vi "Main.vi"(10 "Monedas Subpanel":refnum<vi>, 11 "Module Admin":refnum<class "Delacor_lib_QMH_Module Admin.lvclass">) -> ()   [LabVIEW 2020, in "Monedas.lvlib"]
doc: "This template is based off of the Queued Message Handler design pattern and the Queued Message Handler project template that ships with LabVIEW.\n\nThe main difference is that the queue is private to this module and communication between modules is performed via Broadcast and Request events.\n\nRequest events are wrapped in public API methods and are handled in the Event Handling Loop (EHL) of this VI. Any module can register for Broadcast events sent by this module. The EHL generates messages based on user interface actions.\n\nThe Message Handling Loop (MHL) processes messages generated by the EHL, or by other messages. The messages are string values, so new messages can be added easily to the Message Cases case structure in the MHL. Each message cluster can also provide an optional value for Message Data, which is a variant that can be converted to whatever message-specific data is required.\n_____\nBased on Delacor QMH Project Template 5.0.0.82."
uses:
  Monedas.lvlib
  <vilib>/Delacor/Delacor QMH/Libraries/Module Admin_class/Delacor_lib_QMH_Module Admin.lvclass
  Module Data--cluster.ctl
  Stop Argument--cluster.ctl
  <vilib>/Delacor/Delacor QMH/Libraries/Message Queue_class/Delacor_lib_QMH_Message Queue.lvclass/Delacor_lib_QMH_Message Queue.ctl
  <vilib>/Delacor/Delacor QMH/Libraries/Module Admin_class/Delacor_lib_QMH_Module Admin.lvclass/Delacor_lib_QMH_Module Admin.ctl
  Coin pressed Argument--cluster.ctl
  Set coin values Argument--cluster.ctl
  Reset credit to 0 Argument--cluster.ctl
  Ask if credit Argument--cluster.ctl
  Ask if credit (Reply Payload)--cluster.ctl
  <vilib>/Utility/miscctls.llb/LVPointTypeDef.ctl
  <vilib>/Delacor/Delacor QMH/Libraries/Message Queue_class/Delacor_lib_QMH_Enqueue Message (Single).vi
  <vilib>/Delacor/Delacor QMH/Libraries/Module Admin_class/Delacor_lib_QMH_Get External Launch.vi
  <vilib>/Utility/error.llb/Error Cluster From Error Code.vi
  <vilib>/ErrorRing/Error Ring.xnode
  <vilib>/Delacor/Delacor QMH/Libraries/Message Queue_class/Delacor_lib_QMH_Message Queue.lvclass
  Mensajes/Mensajes.lvlib
panel:
  out "Status":string
  in  "Monedas":cluster{"1":bool, "2":bool, "3":bool, "4":bool}
  out "error out":errorcluster
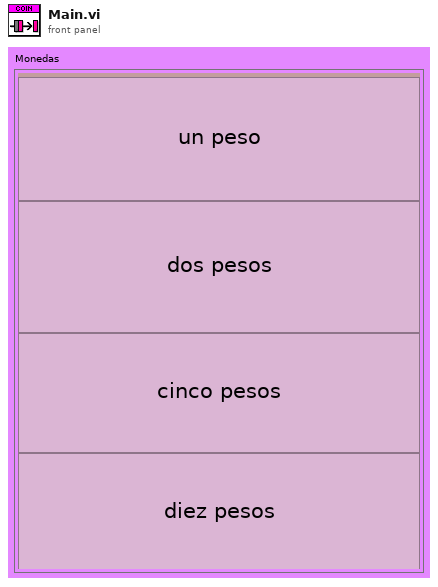
[diagram p1: front panel]
types:
  T1 = typedef "Monedas.lvlib/Request Events--cluster.ctl" = cluster{"Stop Module":refnum<user-event>, "Show Panel":refnum<user-event>, "Hide Panel":refnum<user-event>, "Get Module Execution Status":refnum<user-event>, "Show Diagram":refnum<user-event>, "Coin pressed":refnum<user-event>, "Set coin values":refnum<user-event>, "Request credit":refnum<user-event>, "Reset credit to 0":refnum<user-event>, "Ask if credit":refnum<user-event>}
  T2 = typedef "Monedas.lvlib/Module Data--cluster.ctl" = cluster{"Status":string, "Credit":dbl, "Refs":cluster{"Ref 1":refnum<vi>, "Ref 2":refnum<vi>, "Ref 3":refnum<vi>, "Ref 4":refnum<vi>}, "Coins":cluster{"Boolean Text":string, "Value":i32}[]}
  T3 = enum32{"invalid lock state", "Not Locked", "Locked (No Password)", "Password-protected"}
  T4 = typedef "Monedas.lvlib/Stop Argument--cluster.ctl" = cluster{"Origin":string, "Exit via Stop Module Req?":bool, "Wait for Module to stop?":bool}
  T5 = typedef "Monedas.lvlib/Coin pressed Argument--cluster.ctl" = cluster{"Coin Number":i32}
  T6 = typedef "Monedas.lvlib/Set coin values Argument--cluster.ctl" = cluster{"Coins":cluster{"Boolean Text":string, "Value":i32}[]}
  T7 = typedef "Monedas.lvlib/Reset credit to 0 Argument--cluster.ctl" = cluster{"Boolean":bool}
  T8 = typedef "Monedas.lvlib/Ask if credit Argument--cluster.ctl" = cluster{"Wait Notifier":refnum<notifier>, "wait for reply":bool}
  T9 = typedef "LVPointTypeDef.ctl" = cluster{"Horizontal":i16, "Vertical":i16}
  T10 = enum32{"Invalid", "Standard", "Closed", "Hidden", "Minimized", "Maximized"}
  T11 = typedef "Monedas.lvlib/Ask if credit (Reply Payload)--cluster.ctl" = cluster{"Credit":dbl, "Ask if credit_error":errorcluster}
  T12 = cluster{"Ref 1":refnum<vi>, "Ref 2":refnum<vi>, "Ref 3":refnum<vi>, "Ref 4":refnum<vi>}
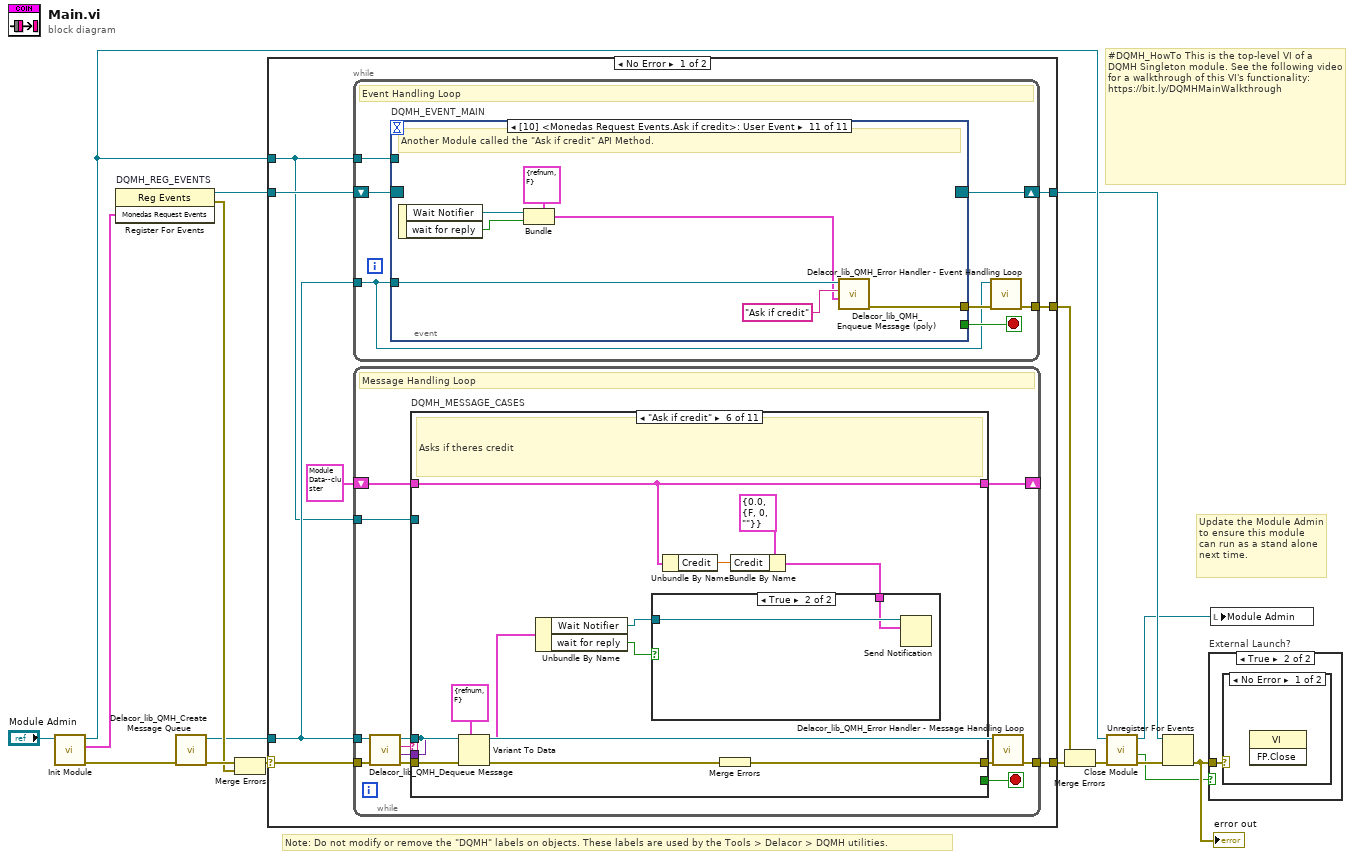
[diagram p0: block diagram]
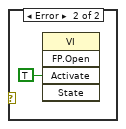
[diagram p3: hidden frame]
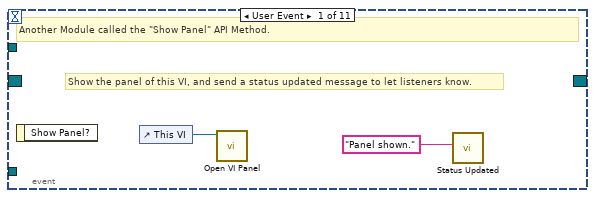
[diagram p4: hidden frame]
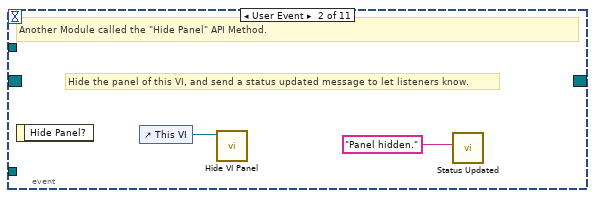
[diagram p5: hidden frame]
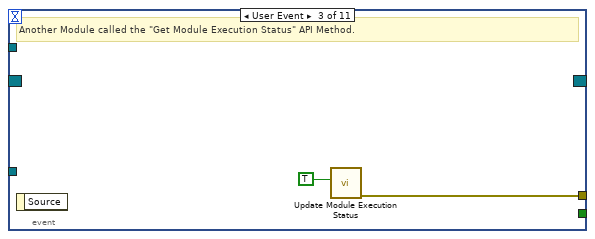
[diagram p6: hidden frame]
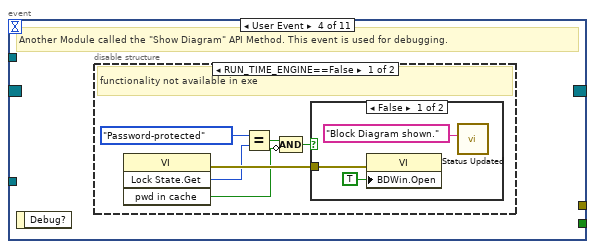
[diagram p7: hidden frame]
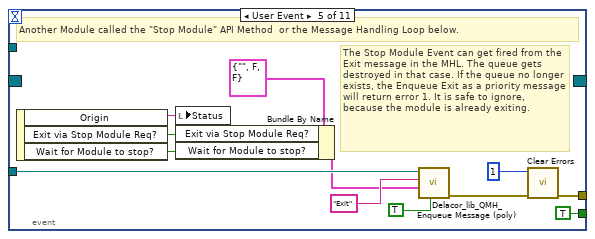
[diagram p10: hidden frame]
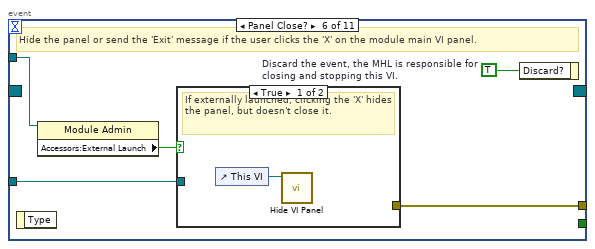
[diagram p11: hidden frame]
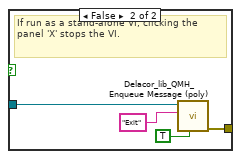
[diagram p12: hidden frame]
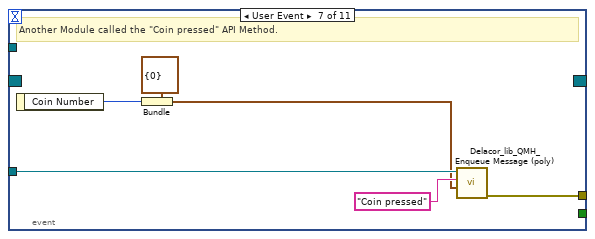
[diagram p13: hidden frame]
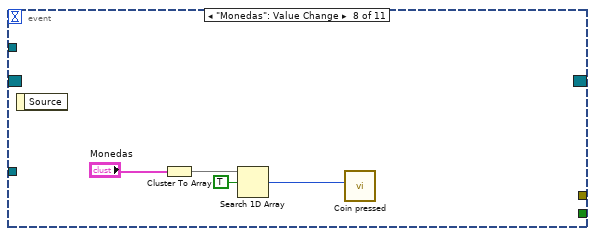
[diagram p14: hidden frame]
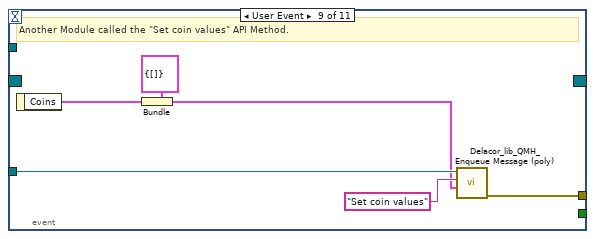
[diagram p15: hidden frame]
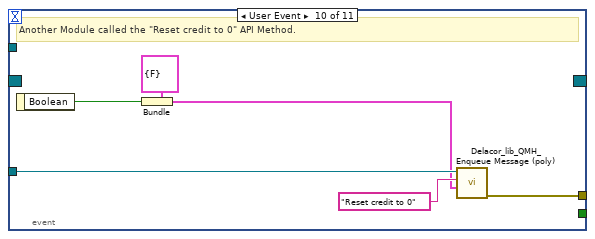
[diagram p16: hidden frame]
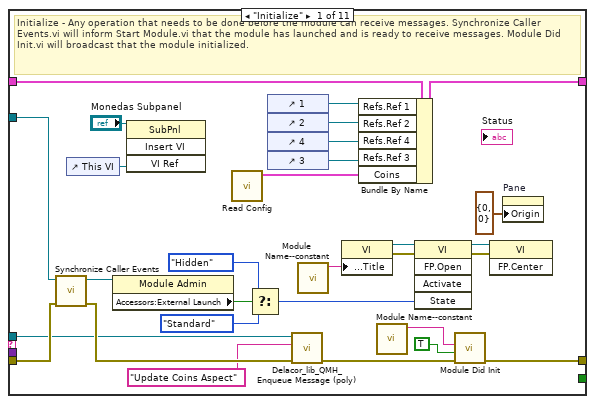
[diagram p17: hidden frame]
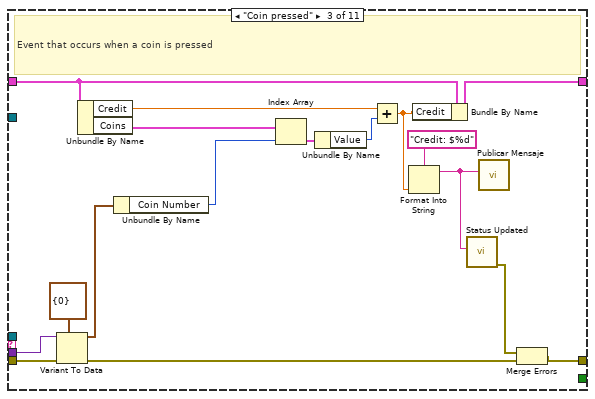
[diagram p19: hidden frame]
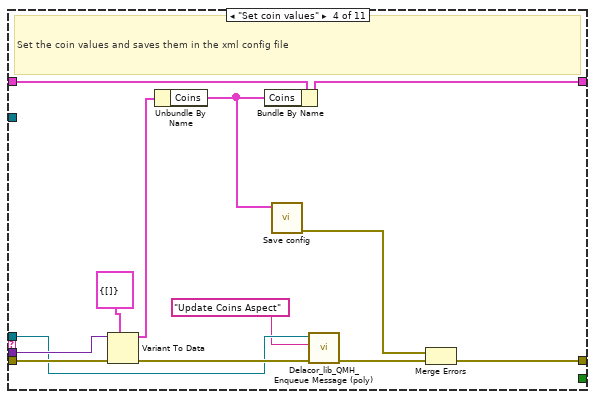
[diagram p20: hidden frame]
diagram:
  # "#DQMH_HowTo This is the top-level VI of a DQMH Singleton module. See the following video for a walkthrough of this VI's functionality: https://bit.ly/DQMHMainWalkthrough"
  # "Note: Do not modify or remove the \"DQMH\" labels on objects. These labels are used by the Tools > Delacor > DQMH utilities."
  # "Update the Module Admin to ensure this module can run as a stand alone next time."
  n1 = call "Init Module.vi"("Singleton Module Admin in"="Module Admin") -> ("error out"=w16:errorcluster, "Monedas Request Events"=w5:T1, "Singleton Module Admin out"=w8:refnum<class "Delacor_lib_QMH_Module Admin.lvclass">)  [unwired: 8 in]
  n2 = register-events "DQMH_REG_EVENTS"(w5) -> (reference out=w6:refnum<event-registration>, error out=w9:errorcluster)  [unwired: 2 in]
  n3 = call <vilib>:"Delacor_lib_QMH_Create Message Queue.vi"("error in (no error)"=w16) -> ("error out"=w11:errorcluster, "Message Queue"=w4:refnum<class "Delacor_lib_QMH_Message Queue.lvclass">)  [unwired: 9 in]
  n4 = Merge Errors(w11, w9) -> (w10:errorcluster)
  n5 = case shown="No Error" w10 {
    selector: w10 -> [w23 w251]
    tunnel: [w25 w250] -> w17
    tunnel: [w22 w256] -> w7
    tunnel: w6 -> [w20 w256]
    tunnel: w4 -> [w19 w249]
    tunnel: [w24 _] -> w14
    tunnel: w8 -> [w18 w252]
    frame No Error {
      n6 = while {
        tunnel: w19 -> [w26]
        shift-right: [w29] -> w22
        shift-left: w20 -> [w30]
        tunnel: [w31] -> w24
        tunnel: w18 -> [w27]
        stop <- w28 stop-if-true
        # "Event Handling Loop"
        n7 = event "DQMH_EVENT_MAIN" shown="[10] <Monedas Request Events.Ask if credit>: User Event" {
          selector: w30 -> [_ _ _ _ _ _ _ _ _ _ _]
          dyn-events: [_ _ _ _ _ _ _ _ _ _ _] -> w29
          timeout: _ -> [_ _ _ _ _ _ _ _ _ _ _]
          tunnel: [_ _ _ _ TRUE ("Discard?") _ _ _ _ _ _] -> w28
          tunnel: w26 -> [_ _ _ _ w55 w62 w75 _ w85 w91 w98]
          tunnel: [_ _ w38 _ w58 w64 w71 _ w80 w86 w92] -> w32
          tunnel: w27 -> [_ _ _ _ _ w61 _ _ _ _ _]
          event User Event {
            # "Show the panel of this VI, and send a status updated message to let listeners know."
            # "Another Module called the \"Show Panel\" API Method."
            n8 = event-data() -> ()  [unwired: 1 in, 1 out]
            n9 = control-ref of="This VI"() -> (w34:refnum<vi>)
            n10 = call "Open VI Panel.vi"("VI"=w34) -> ()  [unwired: 10 in, 1 out]
            n11 = call "Status Updated.vi"("Status"="Panel shown." ("format string")) -> ()  [unwired: 10 in, 1 out]
          }
          event User Event {
            # "Hide the panel of this VI, and send a status updated message to let listeners know."
            # "Another Module called the \"Hide Panel\" API Method."
            n12 = event-data() -> ()  [unwired: 1 in, 1 out]
            n13 = control-ref of="This VI"() -> (w36:refnum<vi>)
            n14 = call "Hide VI Panel.vi"("VI"=w36) -> ()  [unwired: 10 in, 1 out]
            n15 = call "Status Updated.vi"("Status"="Panel hidden." ("format string")) -> ()  [unwired: 10 in, 1 out]
          }
          event User Event {
            # "Another Module called the \"Get Module Execution Status\" API Method."
            n16 = event-data() -> ()  [unwired: 1 in, 1 out]
            n17 = call "Update Module Execution Status.vi"("Running?"=TRUE) -> ("error out"=w38:errorcluster)  [unwired: 10 in]
          }
          event User Event {
            # "Another Module called the \"Show Diagram\" API Method. This event is used for debugging."
            n18 = event-data() -> ()  [unwired: 1 in, 1 out]
            n19 = disable-structure shown="RUN_TIME_ENGINE==False" {
              frame condition #0 (active) {
                # "functionality not available in exe"
                n20 = invoke class="VI" method="Lock State.Get"() -> (error out=w44:errorcluster, "Get Lock State"=w43:T3, "pwd in cache"=w40:bool)  [unwired: 4 in, 1 out]
                n21 = Equal?(x=T3."Password-protected", y=w43) -> (x = y?=w41:bool)
                n22 = Compound Arithmetic op=AND(w41, invert w40) -> (w39:bool)
                n23 = case shown="False" w39 {
                  tunnel: w44 -> [w47 _]
                  frame False {
                    n24 = property class="VI"(error in=w47, "BDWin.Open"=TRUE ("Block Diagram Window:Open")) -> ()  [unwired: 1 in, 2 out]
                    n25 = call "Status Updated.vi"("Status"="Block Diagram shown." ("format string")) -> ()  [unwired: 10 in, 1 out]
                  }
                  frame True {
                    # "Password-protected VI, and the password is not in the cache. Do not show the diagram."
                  }
                }
              }
              frame condition #1 {
              }
            }
          }
          event User Event {
            # "The Stop Module Event can get fired from the Exit message in the MHL. The queue gets destroyed in that case. If the queue no longer exists, the Enqueue Exit as a priority message will return error 1. It is safe to ignore, because the module is already exiting."
            # "Another Module called the \"Stop Module\" API Method  or the Message Handling Loop below."
            n26 = event-data() -> ("Origin"=w54:string, "Exit via Stop Module Req?"=w50:bool, "Wait for Module to stop?"=w49:bool)  [unwired: 1 in]
            n27 = local write "Status"(w54) -> ()
            n28 = Bundle By Name(cluster=T4 {"Origin"="", "Exit via Stop Module Req?"=FALSE, "Wait for Module to stop?"=FALSE} ("Stop Argument"), "Exit via Stop Module Req?"=w50, "Wait for Module to stop?"=w49) -> (w48:T4)
            n29 = call-poly <vilib>:"Delacor_lib_QMH_Enqueue Message (poly).vi"("Priority Message? (F)"=TRUE, "Message Data"=w48, "Message"="Exit", "Message Queue in"=w55) -> ("error out"=w59:errorcluster)  [unwired: 6 in, 1 out]
            n30 = call <vilib>:"Clear Errors.vi"("error in (no error)"=w59, "specific error code to clear (0: all)"=1) -> ("error out"=w58:errorcluster)  [unwired: 4 in, 1 out]
          }
          event Panel Close? {
            w63 = TRUE  # Discard the event, the MHL is responsible for closing and stopping this VI.
            # "Hide the panel or send the 'Exit' message if the user clicks the 'X' on the module main VI panel."
            n31 = event-data() -> ()  [unwired: 1 in, 1 out]
            n32 = property class="Module Admin"(reference=w61) -> ("Accessors:External Launch"=w60:bool)  [unwired: 1 in, 2 out]
            n33 = case shown="True" w60 {
              tunnel: w62 -> [_ w68]
              tunnel: [_ w69] -> w64
              frame True {
                # "If externally launched, clicking the 'X' hides the panel, but doesn't close it."
                n34 = control-ref of="This VI"() -> (w65:refnum<vi>)
                n35 = call "Hide VI Panel.vi"("VI"=w65) -> ()  [unwired: 10 in, 1 out]
              }
              frame False {
                # "If run as a stand-alone VI, clicking the panel 'X' stops the VI."
                n36 = call-poly <vilib>:"Delacor_lib_QMH_Enqueue Message (poly).vi"("Priority Message? (F)"=TRUE, "Message"="Exit", "Message Queue in"=w68) -> ("error out"=w69:errorcluster)  [unwired: 7 in, 1 out]
              }
            }
            n37 = event-data("Discard?"=w63) -> ()  [unwired: 1 in, 1 out]
          }
          event User Event {
            # "Another Module called the \"Coin pressed\" API Method."
            n38 = event-data() -> ("Coin Number"=w70:i32)  [unwired: 1 in]
            n39 = Bundle(cluster=T5 {"Coin Number"=0} ("Coin pressed Argument"), "Coin Number"=w70) -> (w72:T5)
            n40 = call-poly <vilib>:"Delacor_lib_QMH_Enqueue Message (poly).vi"("Message Data"=w72, "Message"="Coin pressed", "Message Queue in"=w75) -> ("error out"=w71:errorcluster)  [unwired: 7 in, 1 out]
          }
          event "Monedas": Value Change {
            n41 = event-data() -> ()  [unwired: 1 in, 1 out]
            n42 = Cluster To Array(cluster="Monedas") -> (array=w78:bool[])
            n43 = Search 1D Array(1D array=w78, element=TRUE) -> (index of element=w77:i32)  [unwired: 1 in]
            n44 = call "Coin pressed.vi"("Coin Number"=w77) -> ()  [unwired: 10 in, 1 out]
          }
          event User Event {
            # "Another Module called the \"Set coin values\" API Method."
            n45 = event-data() -> ("Coins"=w81:cluster{"Boolean Text":string, "Value":i32}[])  [unwired: 1 in]
            n46 = Bundle(cluster=T6 {"Coins"=[]} ("Set coin values Argument"), "Coins"=w81) -> (w82:T6)
            n47 = call-poly <vilib>:"Delacor_lib_QMH_Enqueue Message (poly).vi"("Message Data"=w82, "Message"="Set coin values", "Message Queue in"=w85) -> ("error out"=w80:errorcluster)  [unwired: 7 in, 1 out]
          }
          event User Event {
            # "Another Module called the \"Reset credit to 0\" API Method."
            n48 = event-data() -> ("Boolean"=w87:bool)  [unwired: 1 in]
            n49 = Bundle(cluster=T7 {"Boolean"=FALSE} ("Reset credit to 0 Argument"), "Boolean"=w87) -> (w88:T7)
            n50 = call-poly <vilib>:"Delacor_lib_QMH_Enqueue Message (poly).vi"("Message Data"=w88, "Message"="Reset credit to 0", "Message Queue in"=w91) -> ("error out"=w86:errorcluster)  [unwired: 7 in, 1 out]
          }
          event User Event {
            # "Another Module called the \"Ask if credit\" API Method."
            n51 = event-data() -> ("Wait Notifier"=w94:refnum<notifier>, "wait for reply"=w93:bool)  [unwired: 1 in]
            n52 = Bundle(cluster=T8 {"Wait Notifier"=refnum, "wait for reply"=FALSE} ("Ask if credit Argument"), "Wait Notifier"=w94, "wait for reply"=w93) -> (w95:T8)
            n53 = call-poly <vilib>:"Delacor_lib_QMH_Enqueue Message (poly).vi"("Message Data"=w95, "Message"="Ask if credit", "Message Queue in"=w98) -> ("error out"=w92:errorcluster)  [unwired: 7 in, 1 out]
          }
        }
        n54 = call-dynamic "Delacor_lib_QMH_Error Handler - Event Handling Loop.vi"("error in (no error)"=w32, "Message Queue in"=w26) -> ("dup error in"=w31:errorcluster)  [unwired: 8 in, 1 out]
      }
      n55 = while {
        tunnel: w19 -> [w101]
        shift-right: [w105] -> _
        shift-left: T2 {"Status"="", "Credit"=0.0, "Refs"={"Ref 1"=refnum, "Ref 2"=refnum, "Ref 3"=refnum, "Ref 4"=refnum}, "Coins"=[]} ("Data Cluster") -> [w106]
        tunnel: w23 -> [w109]
        tunnel: [w107] -> w25
        tunnel: w18 -> [w99]
        stop <- w104 stop-if-true
        # "Message Handling Loop"
        n56 = call-dynamic "Delacor_lib_QMH_Dequeue Message.vi"("error in (no error)"=w109, "Message Queue in"=w101) -> ("error out"=w108:errorcluster, "Message Data"=w102:variant, "Message"=w103:string, "Message Queue out"=w100:refnum<class "Delacor_lib_QMH_Message Queue.lvclass">)  [unwired: 6 in]
        n57 = case "DQMH_MESSAGE_CASES" shown="\"Ask if credit\"" w103 {
          selector: w103 -> [_ _ _ _ _ _ _ _ _ _ w236]
          tunnel: w100 -> [w111 _ _ w163 _ _ _ _ w206 w228 _]
          tunnel: w108 -> [w137 w141 w158 w171 w178 w190 w194 w199 w213 w234 w238]
          tunnel: [w135 w141 w144 w160 w176 w181 w194 w199 w209 w231 w239] -> w110
          tunnel: w106 -> [w126 w140 w153 w166 w177 w180 w193 w198 w208 w227 w237]
          tunnel: [w125 w140 w152 w165 w173 w180 w193 w198 w208 w227 w237] -> w105
          tunnel: [_ _ _ _ _ _ _ _ _ w226 _] -> w104
          tunnel: w102 -> [_ _ w156 w169 w175 w188 _ _ w207 w225 _]
          tunnel: w99 -> [w127 _ _ _ _ _ _ _ w205 w220 _]
          frame "Initialize" {
            # "Initialize - Any operation that needs to be done before the module can receive messages. Synchronize Caller Events.vi will inform Start Module.vi that the module has launched and is ready to receive messages. Module Did Init.vi will broadcast that the module initialized."
            n58 = call "Synchronize Caller Events.vi"("error in (no error)"=w137, "Singleton Module Admin in"=w127) -> ("error out"=w136:errorcluster, "Singleton Module Admin out"=w122:refnum<class "Delacor_lib_QMH_Module Admin.lvclass">)  [unwired: 8 in]
            n59 = control-ref of="This VI"() -> (w119:refnum<vi>)
            n60 = property class="Module Admin"(reference=w122) -> ("Accessors:External Launch"=w131:bool)  [unwired: 1 in, 2 out]
            n61 = invoke class="SubPnl" method="Insert VI"(reference="Monedas Subpanel", "VI Ref"=w119) -> ()  [unwired: 2 in, 4 out]
            n62 = call "Read Config.vi"() -> ("value"=w114:cluster{"Boolean Text":string, "Value":i32}[])  [unwired: 9 in, 1 out]
            n63 = Select(t=T10."Hidden" ("State"), s=w131, f=T10."Standard" ("State")) -> (s? t:f=w128:T10)
            n64 = control-ref of="1"() -> (w118:refnum<vi>)
            n65 = control-ref of="2"() -> (w117:refnum<vi>)
            n66 = control-ref of="4"() -> (w116:refnum<vi>)
            n67 = control-ref of="3"() -> (w115:refnum<vi>)
            n68 = call-poly <vilib>:"Delacor_lib_QMH_Enqueue Message (poly).vi"("error in (no error)"=w136, "Message"="Update Coins Aspect", "Message Queue in"=w111) -> ("error out"=w113:errorcluster)  [unwired: 7 in, 1 out]
            n69 = call "Module Name--constant.vi"() -> ("Module Name"=w134:string)  [unwired: 11 in]
            n70 = property class="VI"("Front Panel.Title"=w134) -> (reference out=w133:refnum<vi>, error out=w139:errorcluster)  [unwired: 2 in]
            n71 = Bundle By Name(cluster=w126, "Refs.Ref 1"=w118, "Refs.Ref 2"=w117, "Refs.Ref 4"=w116, "Refs.Ref 3"=w115, "Coins"=w114) -> (w125:T2)
            n72 = call "Module Name--constant.vi"() -> ("Module Name"=w123:string)  [unwired: 11 in]
            n73 = invoke class="VI" method="FP.Open"(reference=w133, error in=w139, "State"=w128) -> (reference out=w132:refnum<vi>, error out=w138:errorcluster)  [unwired: 2 in, 3 out]
            n74 = call "Module Did Init.vi"("error in (no error)"=w113, "Initialized?"=TRUE, "Origin"=w123) -> ("error out"=w135:errorcluster)  [unwired: 8 in]
            n75 = invoke class="VI" method="FP.Center"(reference=w132, error in=w138) -> ()  [unwired: 1 in, 3 out]
            n76 = property on="Pane" class="Pane"("Origin"=T9 {"Horizontal"=0, "Vertical"=0}) -> ()  [unwired: 2 in, 2 out]
          }
          frame "--- Module Specific ---" {
            # "Separator -- The following cases handle messages specific to this Module."
          }
          frame "Coin pressed" {
            # "Event that occurs when a coin is pressed"
            n77 = Variant To Data(error in=w158, type=T5 {"Coin Number"=0} ("Coin pressed Argument"), Variant=w156) -> (data=w154:T5, error out=w157:errorcluster)
            n78 = Unbundle By Name(w153) -> ("Credit"=w147:dbl, "Coins"=w151:cluster{"Boolean Text":string, "Value":i32}[])
            n79 = Unbundle By Name(w154) -> ("Coin Number"=w149:i32)
            n80 = Index Array "Index Array"(array=w151, index=w149) -> (element=w150:cluster{"Boolean Text":string, "Value":i32})
            n81 = Unbundle By Name(w150) -> ("Value"=w148:i32)
            n82 = Add(x=w147, y=w148) -> (x+y=w146:dbl)
            n83 = Format Into String(format string="Credit: $%d", w146) -> (resulting string=w145:string)  [unwired: 2 in, 1 out]
            n84 = Bundle By Name(cluster=w153, "Credit"=w146) -> (w152:T2)
            n85 = call "Status Updated.vi"("Status"=w145) -> ("error out"=w143:errorcluster)  [unwired: 10 in]
            n86 = call "Publicar Mensaje.vi"("Mensaje"=w145) -> ()  [unwired: 10 in, 1 out]
            n87 = Merge Errors(w143, w157) -> (w144:errorcluster)
          }
          frame "Set coin values" {
            # "Set the coin values and saves them in the xml config file"
            n88 = Variant To Data(error in=w171, type=T6 {"Coins"=[]} ("Set coin values Argument"), Variant=w169) -> (data=w167:T6, error out=w170:errorcluster)
            n89 = Unbundle By Name(w167) -> ("Coins"=w161:cluster{"Boolean Text":string, "Value":i32}[])
            n90 = Bundle By Name(cluster=w166, "Coins"=w161) -> (w165:T2)
            n91 = call "Save config.vi"("Coins"=w161) -> ("error out"=w159:errorcluster)  [unwired: 10 in]
            n92 = call-poly <vilib>:"Delacor_lib_QMH_Enqueue Message (poly).vi"("error in (no error)"=w170, "Message"="Update Coins Aspect", "Message Queue in"=w163) -> ("error out"=w164:errorcluster)  [unwired: 7 in, 1 out]
            n93 = Merge Errors(w159, w164) -> (w160:errorcluster)
          }
          frame "Reset credit to 0" {
            # "Resets the credit to 0"
            n94 = Variant To Data(error in=w178, type=T7 {"Boolean"=FALSE} ("Reset credit to 0 Argument"), Variant=w175) -> (error out=w176:errorcluster)  [unwired: 1 out]
            n95 = Bundle By Name(cluster=w177, "Credit"=0.0) -> (w173:T2)
          }
          frame "Ask if credit" {
            # "Asks if theres credit"
            n96 = Variant To Data(error in=w190, type=T8 {"Wait Notifier"=refnum, "wait for reply"=FALSE} ("Ask if credit Argument"), Variant=w188) -> (data=w186:T8, error out=w189:errorcluster)
            n97 = Unbundle By Name(w186) -> ("Wait Notifier"=w185:refnum<notifier>, "wait for reply"=w184:bool)
            n98 = Unbundle By Name(w180) -> ("Credit"=w179:dbl)
            n99 = Merge Errors(w189) -> (w181:errorcluster)
            n100 = Bundle By Name(cluster=T11 {"Credit"=0.0, "Ask if credit_error"={"status"=FALSE, "code"=0, "source"=""}} ("Ask if credit (Reply Payload)"), "Credit"=w179) -> (w183:T11)
            n101 = case shown="True" w184 {
              tunnel: w185 -> [_ w192]
              tunnel: w183 -> [_ w191]
              frame False {
              }
              frame True {
                n102 = Send Notification(notification=w191, notifier=w192) -> ()  [unwired: 1 in, 2 out]
              }
            }
          }
          frame "--- Exit and Error Handling---" {
            # "Separator - The following cases handle errors and exit messages."
          }
          frame "Update Coins Aspect" {
            # "Updates the Coin aspect configured in the config menu"
            n103 = Unbundle By Name(w198) -> ("Refs"=w197:T12, "Coins"=w195:cluster{"Boolean Text":string, "Value":i32}[])
            n104 = Cluster To Array(cluster=w197) -> (array=w196:refnum<vi>[])
            n105 = for {
              tunnel: w196 -> [w202] mode=indexing
              tunnel: w195 -> [w201] mode=indexing
              n106 = Unbundle By Name(w201) -> ("Boolean Text"=w200:string)
              n107 = property class="Bool"(reference=w202, "BoolText.Text"=w200) -> ()  [unwired: 1 in, 2 out]
            }
          }
          frame "Error" {
            # "#CodeRecommended - If you ever change the name of this \"Error\" message, you'll need to update the name in the Check Loop Error.vi as well."
            # "#CodeRecommended - If the module is running in standalone mode (External Launch = FALSE), this code will pop up an error dialog and call the 'Exit' message if an error occurs. Add more fine-grained error handling here."
            # "Error - Check the error message data and respond accordingly. This message is sent by the \"Error Handler\" VIs at the end of each loop in this application."
            n108 = property class="Module Admin"(reference=w205) -> ("Accessors:External Launch"=w204:bool)  [unwired: 1 in, 2 out]
            n109 = Variant To Data(error in=w213, type=errorcluster {"status"=FALSE, "code"=0, "source"=""} ("error constant"), Variant=w207) -> (data=w214:errorcluster, error out=w211:errorcluster)
            n110 = call "Module Name--constant.vi"() -> ("Module Name"=w203:string)  [unwired: 11 in]
            n111 = call "Error Reported.vi"("Additional Information"=w203, "Error"=w214) -> ()  [unwired: 9 in, 1 out]
            n112 = case shown="False" w204 {
              tunnel: [w219 _] -> w210
              tunnel: w206 -> [w217 _]
              tunnel: w214 -> [w218 _]
              frame False {
                # "If the module is running standalone, then pop up an error dialog and call the \"Exit\" message."
                n113 = call <vilib>:"Simple Error Handler.vi"("error in (no error)"=w218) -> ()  [unwired: 4 in, 5 out]
                n114 = call-poly <vilib>:"Delacor_lib_QMH_Enqueue Message (poly).vi"("Priority Message? (F)"=TRUE, "Message"="Exit", "Message Queue in"=w217) -> ("error out"=w219:errorcluster)  [unwired: 7 in, 1 out]
              }
              frame True {
                # "If the module was launched externally, calling the Error Reported broadcast VI is the only action performed by the \"Error\" message. The module's caller can then process the error appropriately."
              }
            }
            n115 = Merge Errors(w211, w210) -> (w209:errorcluster)
            n116 = local write "error out"(w209) -> ()
          }
          frame "Exit" {
            w224 = 91  # 91: not all Exit messages will have an argument
            w226 = TRUE  # Stop the VI
            # "Release the message queue reference"
            # "#CodeNeeded - Add any required cleanup code here"
            # "Exit - Exit the application."
            n117 = Variant To Data(error in=w234, type=T4 {"Origin"="", "Exit via Stop Module Req?"=FALSE, "Wait for Module to stop?"=FALSE} ("Stop Argument"), Variant=w225) -> (data=w222:T4, error out=w230:errorcluster)
            n118 = call <vilib>:"Clear Errors.vi"("error in (no error)"=w230, "specific error code to clear (0: all)"=w224) -> ("error out"=w233:errorcluster)  [unwired: 4 in, 1 out]
            n119 = control-ref of="This VI"() -> (w221:refnum<vi>)
            n120 = call-dynamic "Delacor_lib_QMH_Release Message Queue.vi"("error in (no error)"=w233, "Message Queue"=w228) -> ("error out"=w232:errorcluster)  [unwired: 9 in]
            n121 = call "Handle Exit.vi"("Stop Argument"=w222, "Admin in"=w220, "VI reference"=w221) -> ("error out"=w229:errorcluster)  [unwired: 7 in, 1 out]
            n122 = Merge Errors(w232, w229) -> (w231:errorcluster)
          }
          frame Default {
            # "'Default' case only runs if there is a message that isn't defined in any of the other cases.  Output a programming error."
            n123 = call "Module Name--constant.vi"() -> ("Module Name"=w235:string)  [unwired: 11 in]
            n124 = xnode "Error Ring"("parameter 0"=w236, "parameter 1"=w235) -> ("error out"=w240:errorcluster)
            n125 = Merge Errors(w238, w240) -> (w239:errorcluster)
          }
        }
        n126 = call-dynamic "Delacor_lib_QMH_Error Handler - Message Handling Loop.vi"("error in (no error)"=w110, "Message Queue in"=w100) -> ("dup error in"=w107:errorcluster)  [unwired: 8 in, 1 out]
      }
    }
    frame Error {
      # "Synchronize Caller Events.vi will inform Start Module.vi that the module has launched and will let the code calling Start Module.vi register for broadcasts and would permit the caller receive the broadcast that an error occurred at launch time."
      n127 = call-dynamic "Delacor_lib_QMH_Release Message Queue.vi"("error in (no error)"=w251, "Message Queue"=w249) -> ("error out"=w250:errorcluster)  [unwired: 9 in]
      n128 = call "Synchronize Caller Events.vi"("Singleton Module Admin in"=w252) -> ("error out"=w257:errorcluster)  [unwired: 9 in, 1 out]
      n129 = call "Module Name--constant.vi"() -> ("Module Name"=w255:string)  [unwired: 11 in]
      n130 = Format Into String(format string="An error occurred during initialization. %s is no longer running.", w255) -> (resulting string=w253:string)  [unwired: 2 in, 1 out]
      n131 = Merge Errors(w250, w257) -> (w258:errorcluster)
      n132 = call "Error Reported.vi"("Additional Information"=w253, "Error"=w258) -> ()  [unwired: 9 in, 1 out]
    }
  }
  n133 = Merge Errors(w14, w17) -> (w13:errorcluster)
  n134 = call "Close Module.vi"("error in (no error)"=w13, "Module Admin in"=w8) -> ("error out"=w15:errorcluster, "External Launch"=w1:bool, "Module Admin out"=w2:refnum<class "Delacor_lib_QMH_Module Admin.lvclass">)  [unwired: 7 in]
  n135 = Unregister For Events(event registration refnum=w7, error in=w15) -> (error out=w12:errorcluster)
  "error out" <- w12
  n136 = case "External Launch?" shown="True" w1 {
    tunnel: w12 -> [_ w259]
    frame False {
    }
    frame True {
      n137 = case shown="No Error" w259 {
        frame No Error {
          n138 = invoke class="VI" method="FP.Close"() -> ()  [unwired: 3 in, 3 out]
        }
        frame Error {
          n139 = invoke class="VI" method="FP.Open"("Activate"=TRUE ("Activate?")) -> ()  [unwired: 4 in, 5 out]
        }
      }
    }
  }
  n140 = local write "Module Admin"(w2) -> ()
